vi "About.vi"() -> ()   [LabVIEW 2025]
panel:
  in  "BtTancar":bool
  # "dtecnic@jba.es"
  # "www.jba.es"
  # "dcomercial@jba.es"
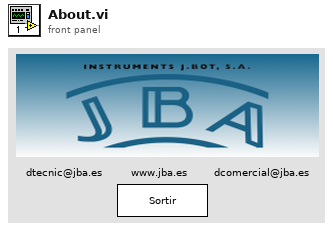
[diagram p1: front panel]
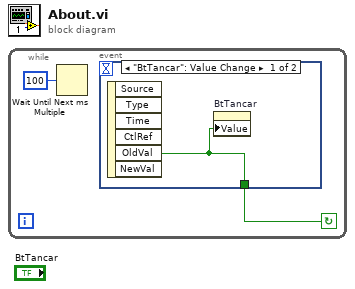
[diagram p0: block diagram]
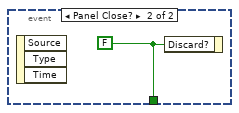
[diagram p2: hidden frame]
diagram:
  n1 = while {
    stop <- w1 continue-if-true
    n2 = Wait Until Next ms Multiple(millisecond multiple=u32 100) -> ()  [unwired: 1 out]
    n3 = event shown="[0] \"BtTancar\": Value Change" {
      selector: _ -> [_ _]
      dyn-events: _ -> [_ _]
      timeout: _ -> [_ _]
      tunnel: [w3 w4] -> w1
      event "BtTancar": Value Change {
        n4 = event-data() -> ("OldVal"=w3:bool)  [unwired: 1 in, 5 out]
        n5 = property on="BtTancar" class="Bool (strict)"("Value"=w3) -> ()  [unwired: 2 in, 2 out]
      }
      event Panel Close? {
        w4 = FALSE ("Discard?")
        n6 = event-data() -> ()  [unwired: 1 in, 3 out]
        n7 = event-data("Discard?"=w4) -> ()  [unwired: 1 in, 1 out]
      }
    }
  }
